vi "Tank Data Global.vi"(0 "Tank Data IN":dbl[](array[numeric]), 1 "Tank Temp Variables":T4, 2 "Speed":dbl[](array[numeric]), 3 "Watlow Present":bool, 4 "Pressure Offsets":dbl[](array[numeric])=[0.0, 0.0, 0.0, 0.0, 0.0, 0.0], 5 "Cal Coefficients":dbl[][](array[numeric]), 6 "Pump Data Mode":T5, 8 "DI23 In":bool, 10 "Read Diagnostics":bool, 11 "Pumps Present":bool[](array[boolean]), 13 "Diagnostics In":dbl[](array[numeric])=[0.0, 0.0, 0.0, 0.0, 0.0, 0.0]) -> (9 "DI23 Out":bool, 14 "Tank Data OUT":dbl[](array[numeric]), 15 "Pump Data":T3={"Voltages"=[0.015201568603515625, 0.00335693359375, 0.003021240234375, 0.12260055541992188, 0.06085968017578125, 0.052234649658203125], "PumpCurrent"=[0.015201568603515625, 0.00335693359375, 0.003021240234375, 0.0, 0.0, 0.0], "Speed"=[0.0, 0.0, 0.0, 0.0, 0.0, 0.0], "ControllerCurrent"=[0.015201568603515625, 0.00335693359375, 0.003021240234375, 0.0, 0.0, 0.0], "Pressure"=[0.015201568603515625, 0.00335693359375, 0.003021240234375, 0.12260055541992188, 0.06085968017578125, 0.052234649658203125], "Flow"=[0.0, 0.0, 0.0, 0.125, 0.0625, 0.0625], "Elapsed Time (Display)"=[0.0, 0.0, 0.0, 0.0, 0.0, 0.0], "Avg Pressure"=0.0, "Avg Speed"=0.0, "Elapsed Time"=[0.0, 0.0, 0.0, 0.0, 0.0, 0.0]} {"Elapsed Time" format="%<%H:%M:%S>t"; "Elapsed Time (Display)" format="%<%H:%M:%S>t"; "Speed" format="%#_4f"; "ControllerCurrent" format="%#.1g"; "Pressure" format="%#.0f"; "Flow" format="%#.0f"; "PumpCurrent" format="%#.1g"; "Voltages" format="%#.0f"}, 17 "Tank Data":T2 {"PS Actual (V):" format="%.2f"; "Temp1" format="%#_2g"; "Temp2" format="%#_2g"}, 18 "Record Time (sec)":dbl, 19 "Auxiliary Data":T1={"Diagnostic Reading"=[0.015201568603515625, 0.00335693359375, 0.003021240234375, 0.12260055541992188, 0.06085968017578125, 0.052234649658203125], "Auxiliary Flow"=[0.015201568603515625, 0.00335693359375, 0.003021240234375, 0.12260055541992188, 0.06085968017578125, 0.052234649658203125]})   [LabVIEW 2019]
uses:
  Type Defs/Pump Data Mode.ctl
  Controls/Tank Temp Variables.ctl
  Controls/Pump Data.ctl
  Controls/Tank Data.ctl
  Type Defs/Auxiliary Data.ctl
  <vilib>/ptbypt/NI_PtbyPt.lvlib
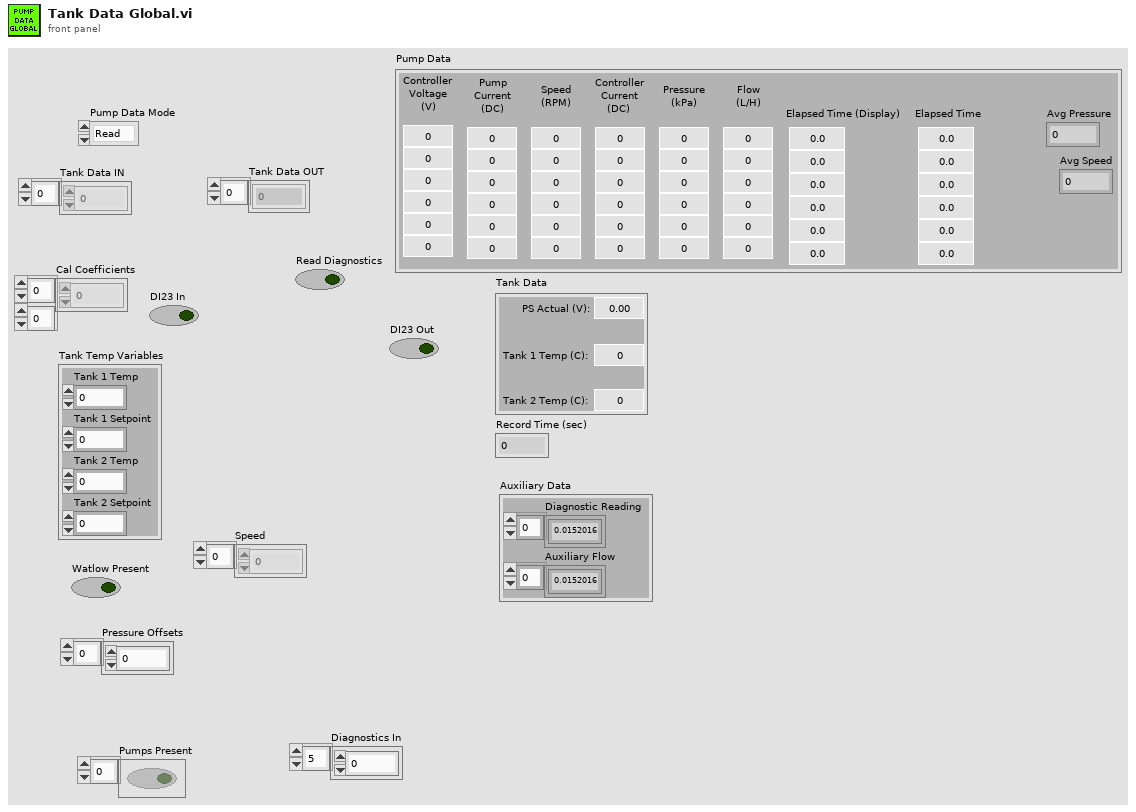
[diagram p1: front panel]
types:
  T1 = typedef "Auxiliary Data.ctl" = cluster{"Diagnostic Reading":dbl[], "Auxiliary Flow":dbl[]}
  T2 = typedef "Tank Data.ctl" = cluster{"PS Actual (V):":dbl, "Temp1":dbl, "Temp2":dbl}
  T3 = typedef "Pump Data.ctl" = cluster{"Voltages":dbl[], "PumpCurrent":dbl[], "Speed":dbl[], "ControllerCurrent":dbl[], "Pressure":dbl[], "Flow":dbl[], "Elapsed Time (Display)":dbl[], "Avg Pressure":dbl, "Avg Speed":dbl, "Elapsed Time":dbl[]}
  T4 = typedef "Tank Temp Variables.ctl" = cluster{"Tank 1 Temp":sgl, "Tank 1 Setpoint":sgl, "Tank 2 Temp":sgl, "Tank 2 Setpoint":sgl}
  T5 = typedef "Pump Data Mode.ctl" = enum16{"Read", "Write Data", "Write Cal", "Write Watlow Data", "Write Pressure Offsets", "Write Pumps Present", "Diagnostic Status", "Write Speed"}
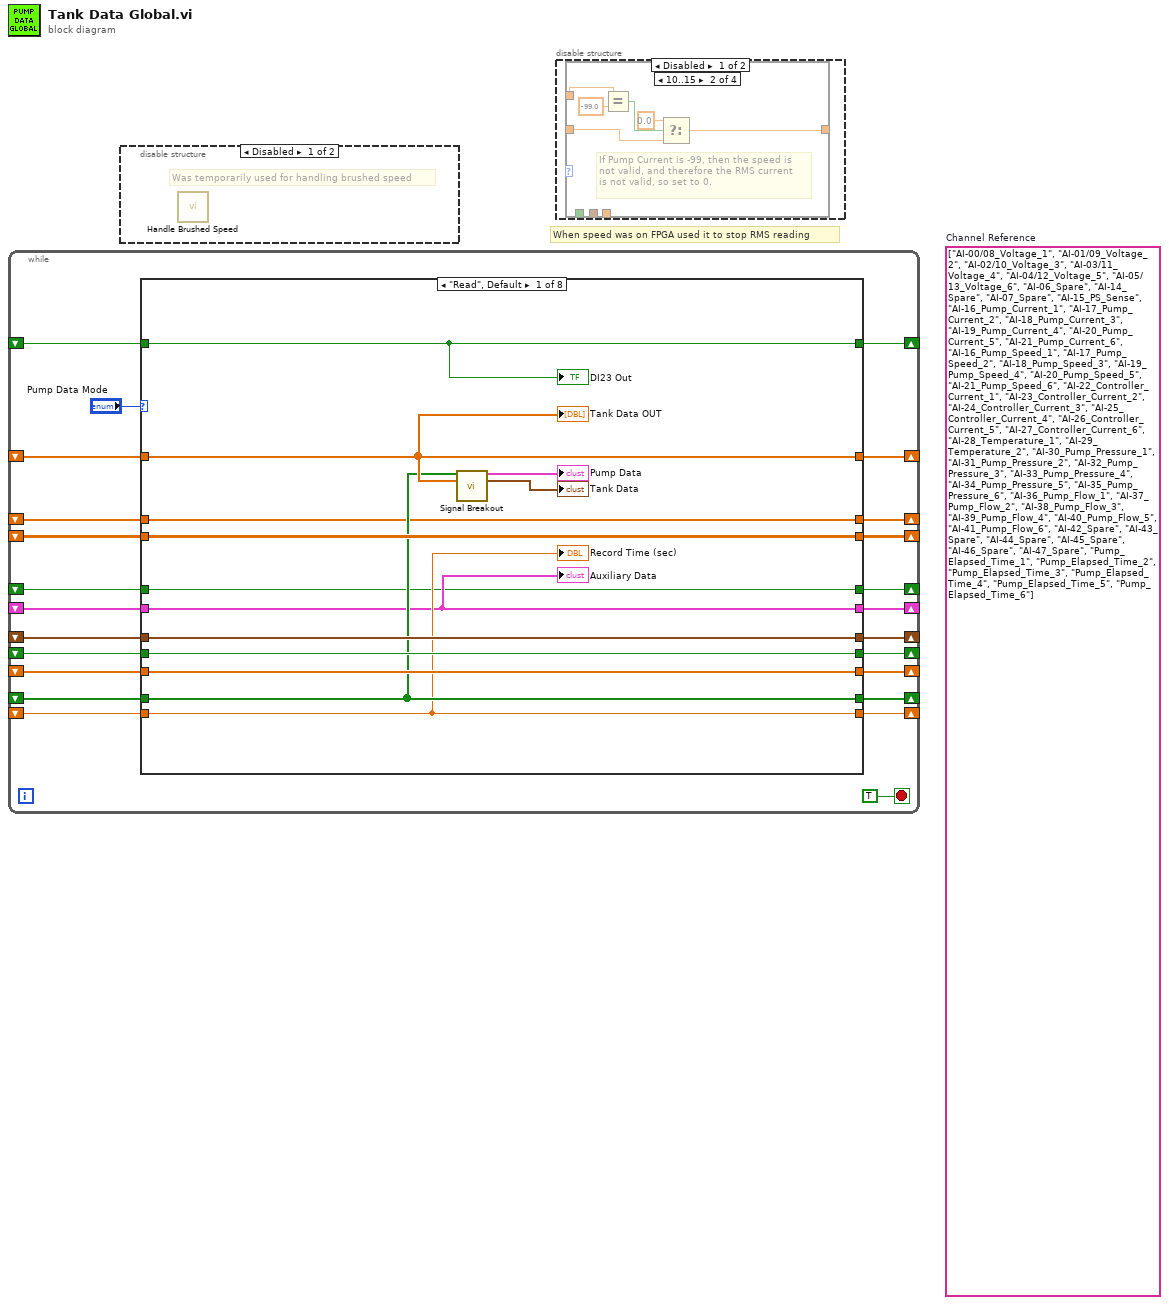
[diagram p0: block diagram]
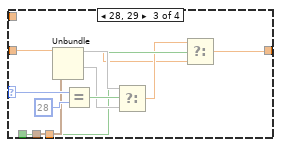
[diagram p3: hidden frame]
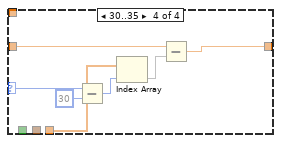
[diagram p4: hidden frame]
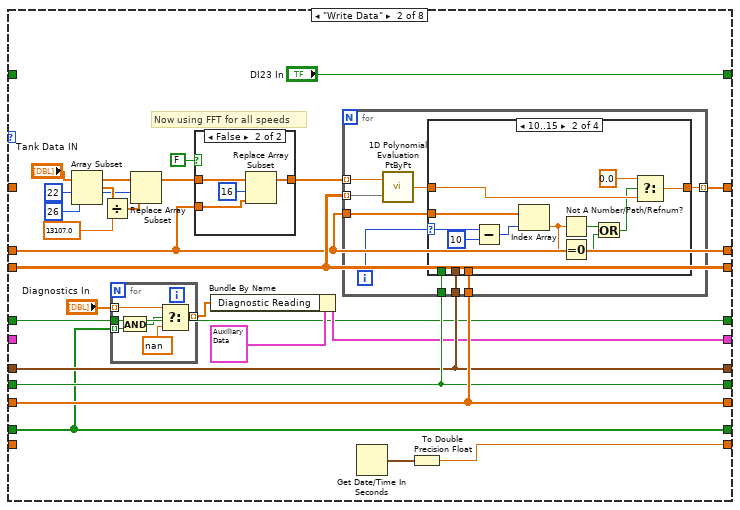
[diagram p7: hidden frame]
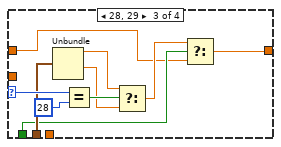
[diagram p10: hidden frame]
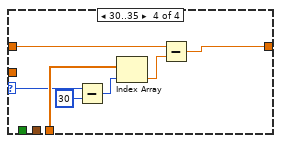
[diagram p11: hidden frame]
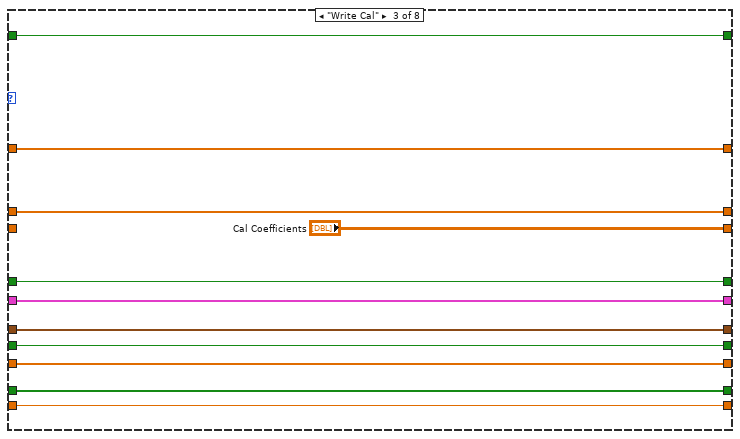
[diagram p12: hidden frame]
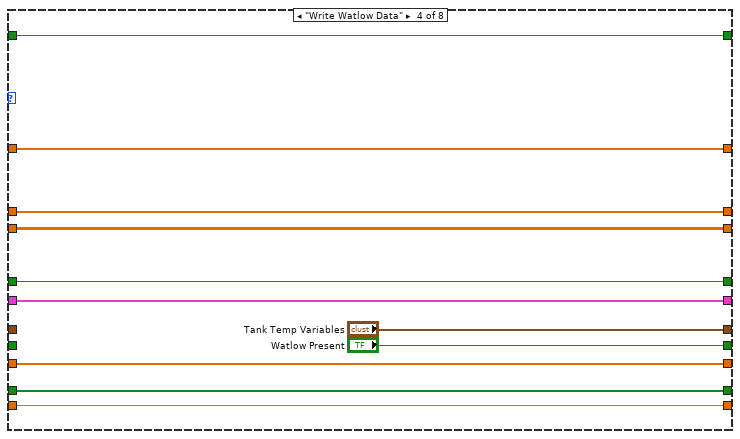
[diagram p13: hidden frame]
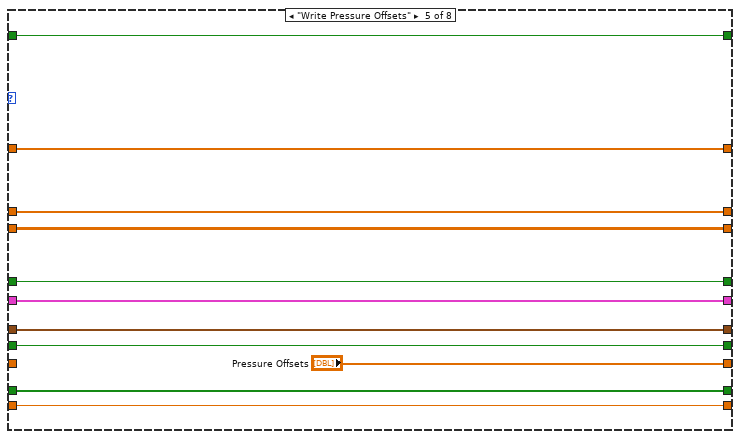
[diagram p14: hidden frame]
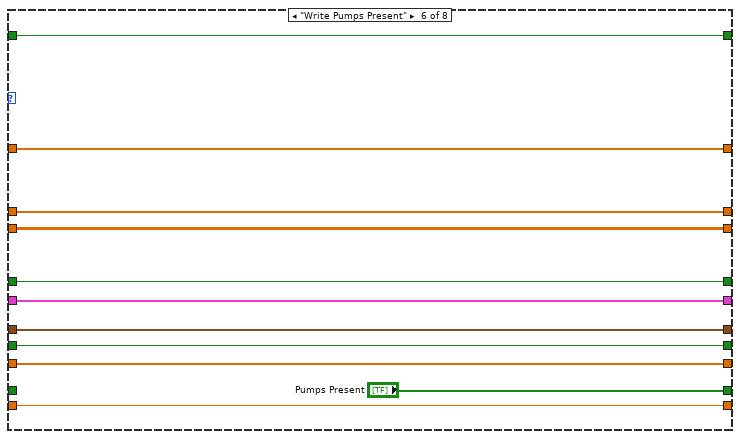
[diagram p15: hidden frame]
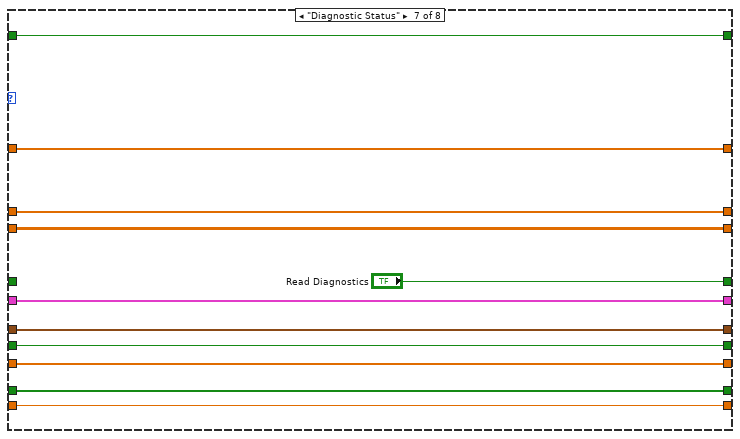
[diagram p16: hidden frame]
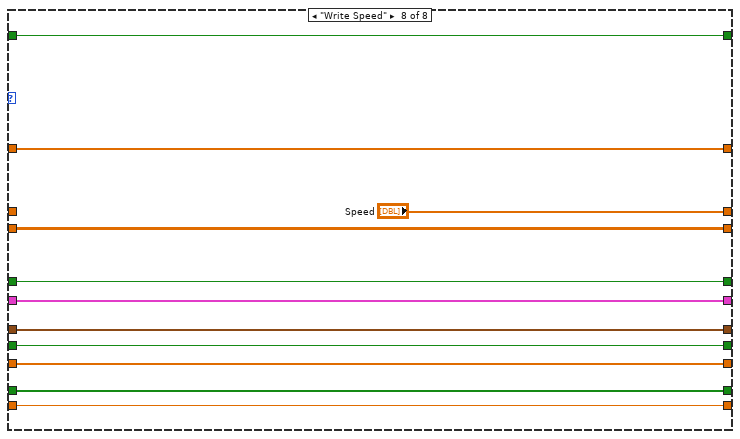
[diagram p17: hidden frame]
diagram:
  (unwired) string[] ["AI-00/08_Voltage_1", "AI-01/09_Voltage_2", "AI-02/10_Voltage_3", "AI-03/11_Voltage_4", "AI-04/12_Voltage_5", "AI-05/13_Voltage_6", "AI-06_Spare", "AI-14_Spare", "AI-07_Spare", "AI-15_PS_Sense", "AI-16_Pump_Current_1", "AI-17_Pump_Current_2", "AI-18_Pump_Current_3", "AI-19_Pump_Current_4", "AI-20_Pump_Current_5", "AI-21_Pump_Current_6", "AI-16_Pump_Speed_1", "AI-17_Pump_Speed_2", "AI-18_Pump_Speed_3", "AI-19_Pump_Speed_4", "AI-20_Pump_Speed_5", "AI-21_Pump_Speed_6", "AI-22_Controller_Current_1", "AI-23_Controller_Current_2", "AI-24_Controller_Current_3", "AI-25_Controller_Current_4", "AI-26_Controller_Current_5", "AI-27_Controller_Current_6", "AI-28_Temperature_1", "AI-29_Temperature_2", "AI-30_Pump_Pressure_1", "AI-31_Pump_Pressure_2", "AI-32_Pump_Pressure_3", "AI-33_Pump_Pressure_4", "AI-34_Pump_Pressure_5", "AI-35_Pump_Pressure_6", "AI-36_Pump_Flow_1", "AI-37_Pump_Flow_2", "AI-38_Pump_Flow_3", "AI-39_Pump_Flow_4", "AI-40_Pump_Flow_5", "AI-41_Pump_Flow_6", "AI-42_Spare", "AI-43_Spare", "AI-44_Spare", "AI-45_Spare", "AI-46_Spare", "AI-47_Spare", "Pump_Elapsed_Time_1", "Pump_Elapsed_Time_2", "Pump_Elapsed_Time_3", "Pump_Elapsed_Time_4", "Pump_Elapsed_Time_5", "Pump_Elapsed_Time_6"]  # Channel Reference
  # "When speed was on FPGA used it to stop RMS reading"
  n1 = while {
    shift-right: [w23] -> _
    shift-left: _ -> [w22]
    shift-right: [w20] -> _
    shift-left: _ -> [w19]
    shift-right: [w18] -> _
    shift-left: _ -> [w17]
    shift-right: [w16] -> _
    shift-left: _ -> [w14]
    shift-right: [w15] -> _
    shift-left: _ -> [w13]
    shift-right: [w12] -> _
    shift-left: _ -> [w11]
    shift-right: [w10] -> _
    shift-left: _ -> [w9]
    shift-right: [w8] -> _
    shift-left: _ -> [w7]
    shift-right: [w6] -> _
    shift-left: _ -> [w5]
    shift-right: [w4] -> _
    shift-left: _ -> [w3]
    shift-right: [w2] -> _
    shift-left: _ -> [w1]
    stop <- TRUE stop-if-true
    n2 = case shown="\"Read\", Default" "Pump Data Mode" {
      tunnel: [w33 w61 w120 w130 w143 w154 w165 w168] -> w23
      tunnel: w22 -> [w33 _ w120 w130 w143 w154 w165 w168]
      tunnel: [w37 w60 "Cal Coefficients" w132 w142 w153 w164 w176] -> w20
      tunnel: w19 -> [w37 w60 _ w132 w142 w153 w164 w176]
      tunnel: [w36 w53 w119 w131 "Pressure Offsets" w150 w160 w171] -> w18
      tunnel: w17 -> [w36 w53 w119 w131 _ w150 w160 w171]
      tunnel: [w35 w51 w118 "Tank Temp Variables" w140 w152 w162 w173] -> w16
      tunnel: [w34 w52 w117 "Watlow Present" w139 w151 w161 w172] -> w15
      tunnel: w14 -> [w35 w51 w118 _ w140 w152 w162 w173]
      tunnel: w13 -> [w34 w52 w117 _ w139 w151 w161 w172]
      tunnel: [w32 w44 w116 w127 w138 "Pumps Present" w159 w170] -> w12
      tunnel: w11 -> [w32 w44 w116 w127 w138 _ w159 w170]
      tunnel: [w29 w49 w115 w126 w137 w148 w158 w169] -> w10
      tunnel: w9 -> [w29 _ w115 w126 w137 w148 w158 w169]
      tunnel: [w28 w48 w114 w125 w136 w147 w163 w174] -> w8
      tunnel: w7 -> [w28 _ w114 w125 w136 w147 w163 w174]
      tunnel: [w27 w45 w113 w124 w135 w146 "Read Diagnostics" w175] -> w6
      tunnel: w5 -> [w27 w45 w113 w124 w135 w146 _ w175]
      tunnel: [w26 w39 w112 w123 w134 w145 w156 "Speed"] -> w4
      tunnel: w3 -> [w26 w39 w112 w123 w134 w145 w156 _]
      tunnel: [w25 "DI23 In" w111 w122 w133 w144 w155 w166] -> w2
      tunnel: w1 -> [w25 _ w111 w122 w133 w144 w155 w166]
      frame "Read", Default {
        n3 = call "Signal Breakout.vi"("Pumps Enabled"=w32, "Tank Data"=w33) -> ("Pump Data"=→"Pump Data":T3, "Tank Data"=→"Tank Data":T2)  [unwired: 12 in]
        "Tank Data OUT" <- w33
        "Record Time (sec)" <- w29
        "Auxiliary Data" <- w28
        "DI23 Out" <- w25
      }
      frame "Write Data" {
        w56 = 22 ("index")
        # "Now using FFT for all speeds"
        n4 = Array Subset(array="Tank Data IN", index=w56, length=26) -> (w57:dbl[])
        n5 = Divide(x=w57, y=13107.0) -> (x/y=w59:dbl[])
        n6 = for {
          tunnel: "Diagnostics In" -> [w69] mode=indexing
          tunnel: w45 -> [w72]
          tunnel: w44 -> [w71] mode=indexing
          tunnel: [w67] -> w43 mode=indexing
          n7 = And(x=w72, y=w71) -> (x .and. y?=w70:bool)
          n8 = Select(t=w69, s=w70, f=nan) -> (s? t:f=w67:dbl)
        }
        n9 = Replace Array Subset(array="Tank Data IN", new element=w59, index=w56) -> (w42:dbl[])
        n10 = case shown="False" FALSE {
          tunnel: w42 -> [w62 w66]
          tunnel: [w62 w65] -> w41
          tunnel: w39 -> [_ w64]
          frame True {
          }
          frame False {
            n11 = Replace Array Subset(array=w66, new element=w64, index=16) -> (w65:dbl[])
          }
        }
        n12 = Bundle By Name(cluster=T1 {"Diagnostic Reading"=[nan, nan, nan, nan, nan, nan], "Auxiliary Flow"=[nan, nan, nan, nan, nan, nan]} ("Auxiliary Data"), "Diagnostic Reading"=w43) -> (w48:T1)
        n13 = for {
          tunnel: w60 -> [w81] mode=indexing
          tunnel: w41 -> [w77] mode=indexing
          tunnel: [w78] -> w61 mode=indexing
          tunnel: w53 -> [w76]
          tunnel: w52 -> [w75]
          tunnel: w51 -> [w74]
          tunnel: w39 -> [w73]
          i -> [w80]
          n14 = call <vilib>:"1D Polynomial Evaluation PtByPt.vi"("Coefficients: a"=w81, "x"=w77) -> ("y"=w79:dbl)
          n15 = case shown="10..15" w80 {
            selector: w80 -> [_ w89 w103 w109]
            tunnel: w79 -> [w82 w93 w95 w106]
            tunnel: [w82 w91 w94 w104] -> w78
            tunnel: w76 -> [_ _ _ w110]
            tunnel: w75 -> [_ _ w97 _]
            tunnel: w74 -> [_ _ w101 _]
            tunnel: w73 -> [_ w90 _ _]
            frame 0, Default {
            }
            frame 10..15 {
              n16 = Subtract(x=w89, y=10) -> (x-y=w87:i32)
              n17 = Index Array(array=w90, index=w87) -> (element=w86:dbl)
              n18 = Not A Number/Path/Refnum?(number/path/refnum=w86) -> (NaN/Path/Refnum?=w85:bool)
              n19 = Equal To 0?(x=w86) -> (x = 0?=w84:bool)
              n20 = Or(x=w85, y=w84) -> (x .or. y?=w83:bool)
              n21 = Select(t=0.0, s=w83, f=w93) -> (s? t:f=w91:dbl)
            }
            frame 28, 29 {
              n22 = Unbundle(w101) -> ("Tank 1 Temp"=w99:sgl, "Tank 2 Temp"=w98:sgl)  [unwired: 2 out]
              n23 = Equal?(x=w103, y=28) -> (x = y?=w100:bool)
              n24 = Select(t=w99, s=w100, f=w98) -> (s? t:f=w96:sgl)
              n25 = Select(t=w96, s=w97, f=w95) -> (s? t:f=w94:dbl)
            }
            frame 30..35 {
              n26 = Subtract(x=w109, y=30) -> (x-y=w107:i32)
              n27 = Index Array(array=w110, index=w107) -> (element=w105:dbl)
              n28 = Subtract(x=w106, y=w105) -> (x-y=w104:dbl)
            }
          }
        }
        n29 = Get Date/Time In Seconds() -> (seconds since 1Jan1904=w50:timestamp)
        n30 = To Double Precision Float(number=w50) -> (double precision float=w49:dbl)
      }
      frame "Write Cal" {
      }
      frame "Write Watlow Data" {
      }
      frame "Write Pressure Offsets" {
      }
      frame "Write Pumps Present" {
      }
      frame "Diagnostic Status" {
      }
      frame "Write Speed" {
      }
    }
  }
  n31 = disable-structure shown="Disabled" {
    frame Disabled {
      # "Was temporarily used for handling brushed speed"
      n32 = call "Handle Brushed Speed.vi"() -> ()  [unwired: 11 in, 1 out]
    }
    frame Enabled {
    }
  }
  n33 = disable-structure shown="Disabled" {
    frame Disabled {
      n34 = case shown="10..15" {
        selector: _ -> [_ _ w193 w199]
        tunnel: _ -> [w177 w180 w185 w196]
        tunnel: [w177 w178 w184 w194] -> _
        tunnel: _ -> [_ w183 _ _]
        tunnel: _ -> [_ _ _ w200]
        tunnel: _ -> [_ _ w187 _]
        tunnel: _ -> [_ _ w191 _]
        frame 0, Default {
        }
        frame 10..15 {
          # "If Pump Current is -99, then the speed is\nnot valid, and therefore the RMS current\nis not valid, so set to 0."
          n35 = Equal?(x=w183, y=-99.0) -> (x = y?=w181:bool)
          n36 = Select(t=0.0, s=w181, f=w180) -> (s? t:f=w178:dbl)
        }
        frame 28, 29 {
          n37 = Unbundle(w191) -> ("Tank 1 Temp"=w189, "Tank 2 Temp"=w188)  [unwired: 2 out]
          n38 = Equal?(x=w193, y=28) -> (x = y?=w190:bool)
          n39 = Select(t=w189, s=w190, f=w188) -> (s? t:f=w186:dbl)
          n40 = Select(t=w186, s=w187, f=w185) -> (s? t:f=w184:dbl)
        }
        frame 30..35 {
          n41 = Subtract(x=w199, y=30) -> (x-y=w197:i32)
          n42 = Index Array(array=w200, index=w197) -> (element=w195)
          n43 = Subtract(x=w196, y=w195) -> (x-y=w194:dbl)
        }
      }
    }
    frame Enabled {
    }
  }
